vi "GenVelLtdProf.vi"() -> ()   [LabVIEW 2016]
panel:
  out "Signals RY":T1
  in  "No Cycles":u16=3
  in  "Dwell Time [s]":dbl=1.0
  in  "Max Speed [/s]":dbl=5.0
  in  "Travel [deg or mm]":dbl=20.0
  in  "Select Joint No.":T2(ring)=enum."Joint 3"
  out "Joint 4 Graph":dbl[](graph)
  out "Joint 3 Graph":dbl[](graph)
  out "Joint 2 Graph":dbl[](graph)
  out "Joint 1 Graph":dbl[](graph)
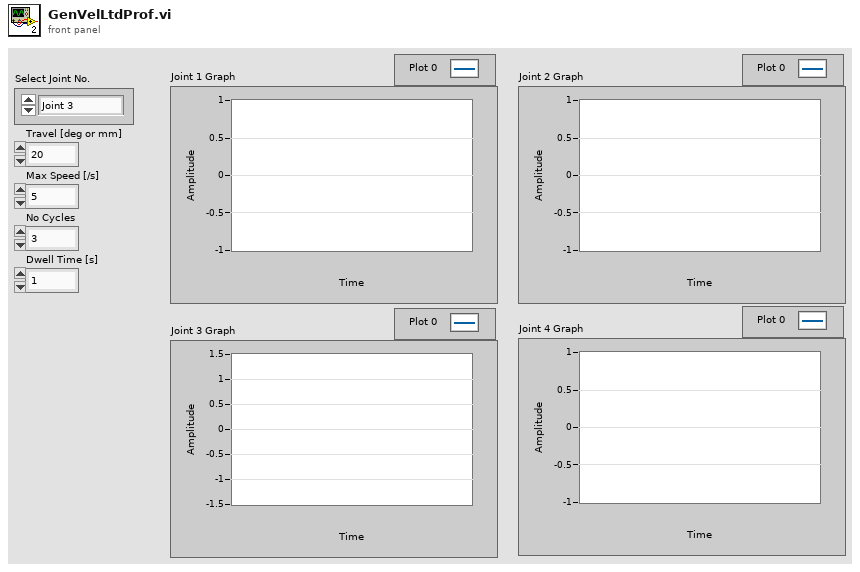
[diagram p1: front panel]
types:
  T1 = cluster{"Ref":cluster{"theta 1 Array":dbl[], "theta 2 Array":dbl[], "d3 Array":dbl[], "theta 4 Array":dbl[]}, "yOut":cluster{"theta 1 Array":dbl[], "theta 2 Array":dbl[], "d3 Array":dbl[], "theta 4 Array":dbl[]}}
  T2 = enum16{"Joint 1", "Joint 2", "Joint 3", "Joint 4"}
  T3 = cluster{"theta 1 Array":dbl[], "theta 2 Array":dbl[], "d3 Array":dbl[], "theta 4 Array":dbl[]}
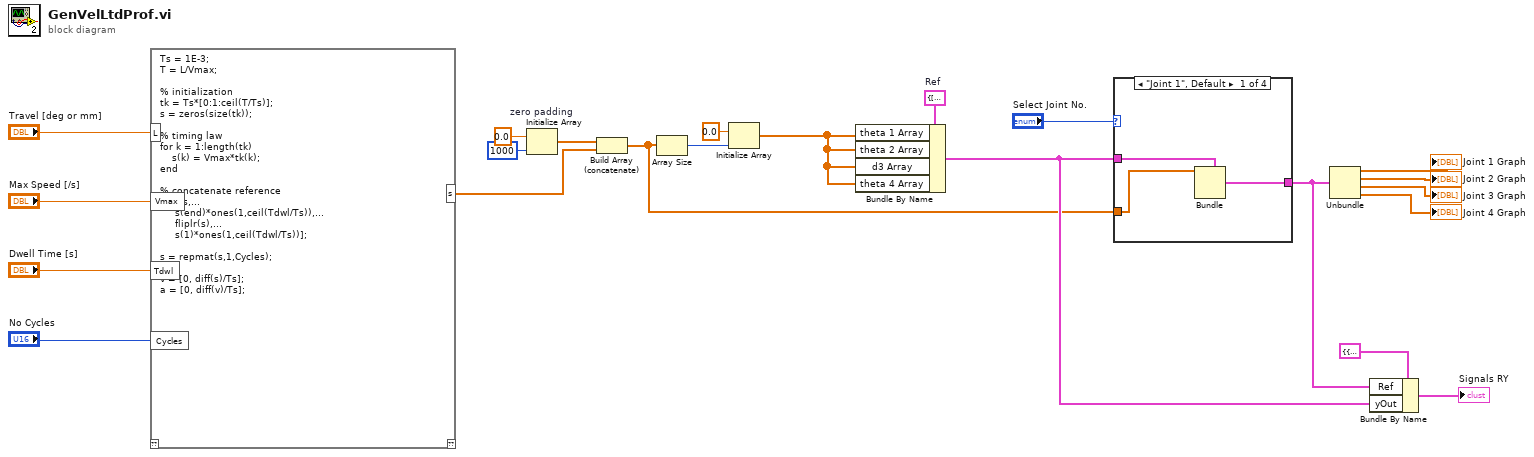
[diagram p0: block diagram]
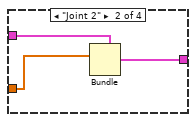
[diagram p2: hidden frame]
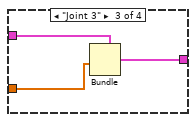
[diagram p3: hidden frame]
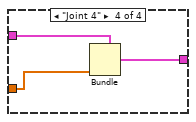
[diagram p4: hidden frame]
diagram:
  w14 = T3 {"theta 1 Array"=[], "theta 2 Array"=[], "d3 Array"=[], "theta 4 Array"=[]}  # Ref
  n1 = script code="Ts = 1E-3;\nT = L/Vmax;\n\n% initialization\ntk = Ts*[0:1:ceil(T/Ts)];\ns = zeros(size(tk));\n\n% timing law\nfor k = 1:length(tk) \n    s(k) = Vmax*tk(k);\nend\n\n% concatenate reference\ns = [s,...\n     s(end)*ones(1,ceil(Tdwl/Ts)),...\n     fliplr(s),...\n     s(1)*ones(1,ceil(Tdwl/Ts))];\n\ns = repmat(s,1,Cycles);\n\nv = [0, diff(s)/Ts];\na = [0, diff(v)/Ts];"("L"="Travel [deg or mm]", "Vmax"="Max Speed [/s]", "Tdwl"="Dwell Time [s]", "Cycles"="No Cycles") -> ("s"=w2:dbl[])  [unwired: 1 in, 1 out]
  n2 = Initialize Array "zero padding"(0.0 ("element"), 1000 ("dimension size")) -> (w3:dbl[])
  n3 = Build Array (concatenate)(w3, w2) -> (w1:dbl[])
  n4 = Array Size(array=w1) -> (size(s)=w18:i32)
  n5 = Initialize Array(0.0 ("element"), w18) -> (w16:dbl[])
  n6 = Bundle By Name(cluster=w14, "theta 1 Array"=w16, "theta 2 Array"=w16, "d3 Array"=w16, "theta 4 Array"=w16) -> (w8:T3)
  n7 = case shown="\"Joint 1\", Default" "Select Joint No." {
    tunnel: w8 -> [w25 w28 w31 w34]
    tunnel: w1 -> [w24 w27 w30 w33]
    tunnel: [w23 w26 w29 w32] -> w9
    frame "Joint 1", Default {
      n8 = Bundle(cluster=w25, "theta 1 Array"=w24) -> (w23:T3)  [unwired: 3 in]
    }
    frame "Joint 2" {
      n9 = Bundle(cluster=w28, "theta 2 Array"=w27) -> (w26:T3)  [unwired: 3 in]
    }
    frame "Joint 3" {
      n10 = Bundle(cluster=w31, "d3 Array"=w30) -> (w29:T3)  [unwired: 3 in]
    }
    frame "Joint 4" {
      n11 = Bundle(cluster=w34, "theta 4 Array"=w33) -> (w32:T3)  [unwired: 3 in]
    }
  }
  n12 = Unbundle(w9) -> ("theta 1 Array"=→"Joint 1 Graph":dbl[], "theta 2 Array"=→"Joint 2 Graph":dbl[], "d3 Array"=→"Joint 3 Graph":dbl[], "theta 4 Array"=→"Joint 4 Graph":dbl[])
  n13 = Bundle By Name(cluster=T1 {"Ref"={"theta 1 Array"=[], "theta 2 Array"=[], "d3 Array"=[], "theta 4 Array"=[]}, "yOut"={"theta 1 Array"=[], "theta 2 Array"=[], "d3 Array"=[], "theta 4 Array"=[]}} ("Track RY Signals"), "Ref"=w9, "yOut"=w8) -> (→"Signals RY":T1)
